vi "HV_Onstate_Single.vi"(8 "On/Off":string(combo), 11 "Channel":string) -> (3 "standard output":string)   [LabVIEW 2018]
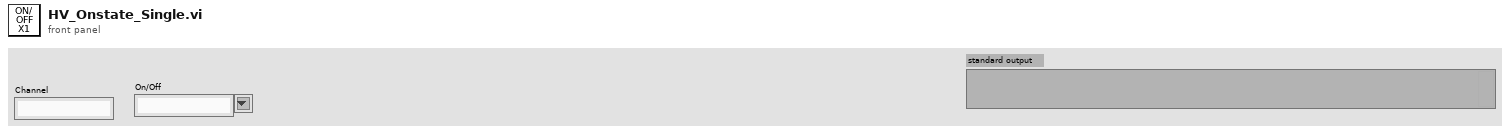
[diagram p1: front panel]
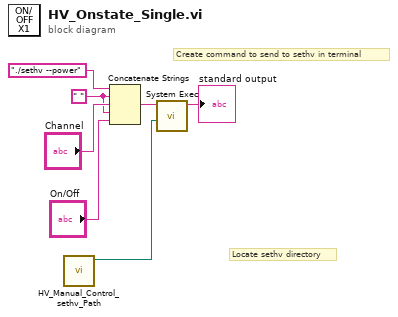
[diagram p0: block diagram]
diagram:
  w4 = " " ("string")
  # "Locate sethv directory"
  # "Create command to send to sethv in terminal"
  n1 = call "HV_Manual_Control_sethv_Path.vi"() -> ("sethv filepath"=w1:path)  [unwired: 11 in]
  n2 = Concatenate Strings("./sethv --power" ("string"), w4, "Channel", w4, "On/Off") -> (w7:string)
  n3 = call <vilib>:"System Exec.vi"("working directory"=w1, "command line"=w7) -> ("standard output"=→"standard output":string)  [unwired: 6 in, 3 out]
